vi "Run.vi"   [LabVIEW 2016]
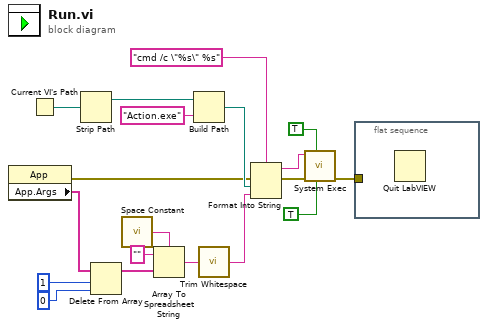
[diagram p0: block diagram]
diagram:
  n1 = property class="App"() -> (error out=w4:errorcluster, "App.Args"=w14:string[])  [unwired: 2 in, 1 out]
  n2 = Current VI's Path() -> (path=w9:path)
  n3 = Strip Path(path=w9) -> (stripped path=w8:path)  [unwired: 1 out]
  n4 = Delete From Array(array=w14, length=1, index=0) -> (array with subset deleted=w13:string[])  [unwired: 1 out]
  n5 = call <vilib>:"Space Constant.vi"() -> ("String"=w18:string)
  n6 = Array To Spreadsheet String(delimiter (Tab)=w18, array=w13, 3:"" ("format string")) -> (spreadsheet string=w15:string)
  n7 = Build Path(base path=w8, name or relative path="Action.exe") -> (appended path=w5:path)
  n8 = call <vilib>:"Trim Whitespace.vi"("string"=w15) -> ("trimmed string"=w3:string)  [unwired: 1 in]
  n9 = Format Into String(format string="cmd /c \"%s\" %s", error in=w4, w5, w3) -> (resulting string=w17:string, error out=w10:errorcluster)  [unwired: 1 in]
  n10 = call <vilib>:"System Exec.vi"("run minimized? (F)"=TRUE, "wait until completion? (T)"=TRUE, "error in (no error)"=w10, "command line"=w17) -> ("error out"=w1:errorcluster)  [unwired: 4 in, 3 out]
  n11 = flat-sequence {
    tunnel: w1 -> [_]
    frame #0 {
      n12 = Quit LabVIEW() -> ()  [unwired: 1 in]
    }
  }
